vi "e.gate HighSpeedPort CodeDataType.vi"(8 "error in (no error)":errorcluster, 9 "Precision":i32, 10 "Value":dbl, 11 "TransferDataType":T1) -> (0 "error out":errorcluster, 1 "ByteCount":i32, 2 "DataTypeString":string, 3 "Binary data out":u8[](array[numeric]))   [LabVIEW 2016]
doc: "This vi codes a numeric value to a binary array with the right data type.\nData types are coded with fixed indexes.\n\nAlso some other useful information's are available."
uses:
  e.gate Data Type.ctl
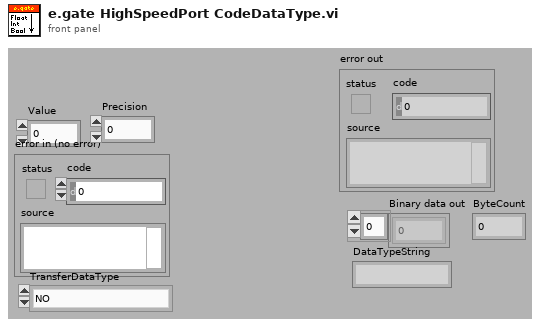
[diagram p1: front panel]
types:
  T1 = typedef "e.gate Data Type.ctl" = enum16{"NO", "BOOL", "SINT8", "USINT8", "SINT16", "USINT16", "SINT32", "USINT32", "FLOAT", "SET8", "SET16", "SET32", "DOUBLE", "SINT64", "USINT64", "SET64"}
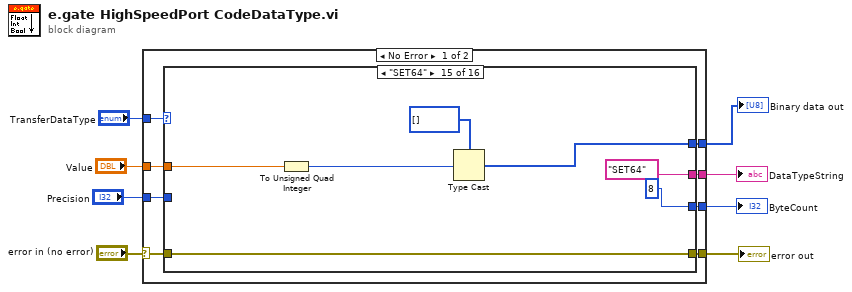
[diagram p0: block diagram]
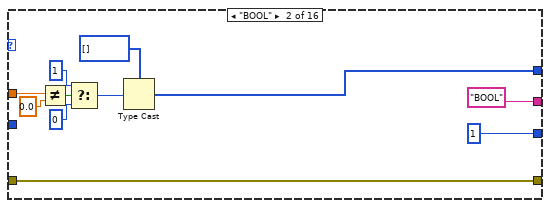
[diagram p3: hidden frame]
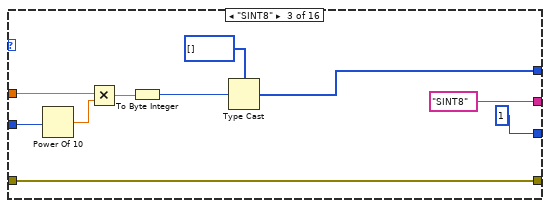
[diagram p4: hidden frame]
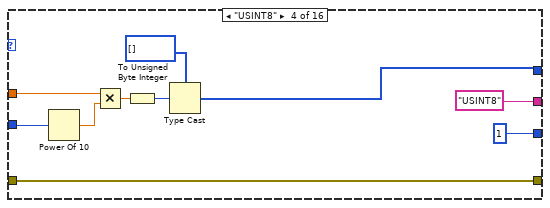
[diagram p5: hidden frame]
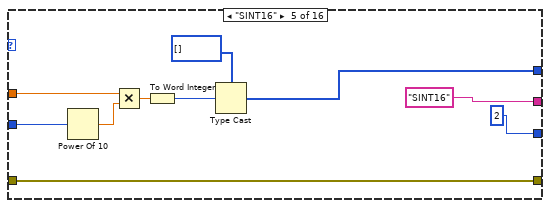
[diagram p6: hidden frame]
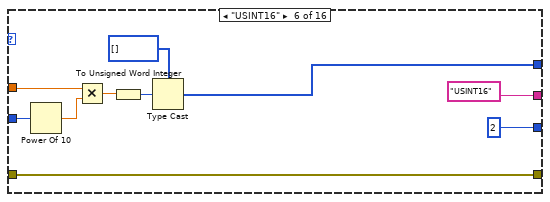
[diagram p7: hidden frame]
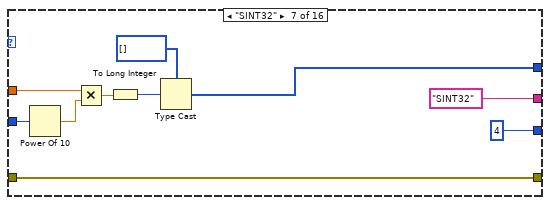
[diagram p8: hidden frame]
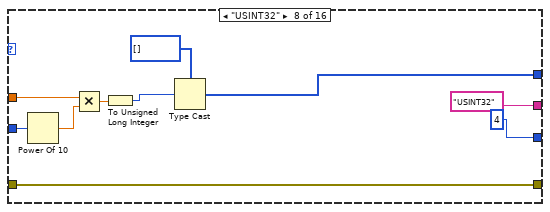
[diagram p9: hidden frame]
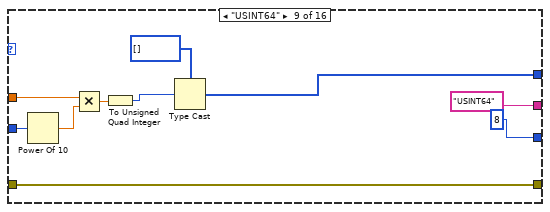
[diagram p10: hidden frame]
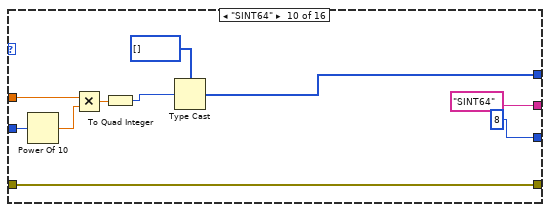
[diagram p11: hidden frame]
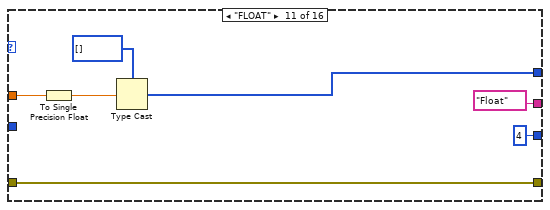
[diagram p12: hidden frame]
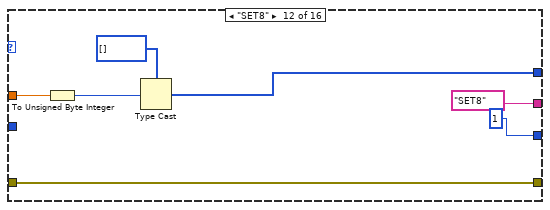
[diagram p13: hidden frame]
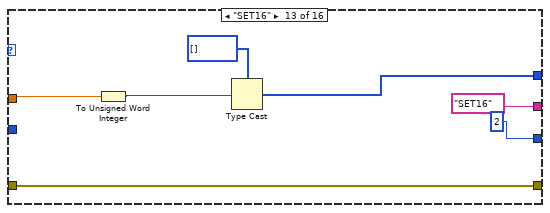
[diagram p14: hidden frame]
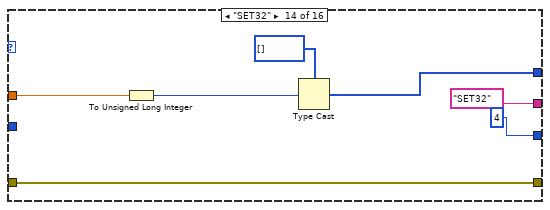
[diagram p15: hidden frame]
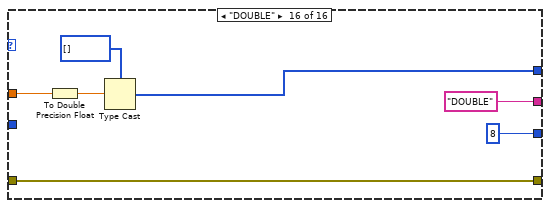
[diagram p16: hidden frame]
diagram:
  n1 = case shown="No Error" "error in (no error)" {
    selector: "error in (no error)" -> [w10 w151]
    tunnel: [w16 w151] -> w8
    tunnel: [w15 _] -> w7
    tunnel: [w14 _] -> w6
    tunnel: "TransferDataType" -> [w13 _]
    tunnel: "Value" -> [w12 _]
    tunnel: [w11 _] -> w4
    tunnel: "Precision" -> [w9 _]
    frame No Error {
      n2 = case shown="\"SET64\"" w13 {
        tunnel: [_ "BOOL" "SINT8" "USINT8" "SINT16" "USINT16" "SINT32" "USINT32" "USINT64" "SINT64" "Float" "SET8" "SET16" "SET32" "SET64" "DOUBLE"] -> w14
        tunnel: w12 -> [_ w23 w31 w41 w51 w61 w71 w81 w91 w101 w113 w119 w123 w130 w137 w148]
        tunnel: [_ i16 1 ("Precision") 1 1 ("Precision") 2 ("Precision") 2 ("Precision") 4 ("Precision") 4 ("Precision") 8 ("Precision") 8 ("Precision") 4 ("Precision") 1 ("Precision") 2 ("Precision") 4 ("Precision") 8 ("Precision") i16 8 ("Precision")] -> w15
        tunnel: [_ w18 w35 w45 w55 w64 w74 w84 w94 w104 w109 w116 w125 w132 w139 w144] -> w11
        tunnel: w10 -> [w17 w21 w34 w44 w54 w66 w76 w86 w96 w106 w112 w120 w127 w134 w141 w147]
        tunnel: [w17 w21 w34 w44 w54 w66 w76 w86 w96 w106 w112 w120 w127 w134 w141 w147] -> w16
        tunnel: w9 -> [_ _ w33 w42 w52 w62 w72 w82 w92 w102 _ _ _ _ _ _]
        frame "NO", Default {
        }
        frame "BOOL" {
          n3 = Not Equal?(x=w23, y=0.0) -> (x != y?=w24:bool)
          n4 = Select(t=u8 1, s=w24, f=u8 0) -> (s? t:f=w20:u8)
          n5 = Type Cast(type=u8[] [] ("Binary data out"), x=w20) -> (*(type *) &x=w18:u8[])
        }
        frame "SINT8" {
          n6 = Power Of 10(x=w33) -> (10^x=w32:dbl)
          n7 = Multiply(x=w31, y=w32) -> (x*y=w30:dbl)
          n8 = To Byte Integer(number=w30) -> (8bit integer=w29:i8)
          n9 = Type Cast(type=u8[] [] ("Binary data out"), x=w29) -> (*(type *) &x=w35:u8[])
        }
        frame "USINT8" {
          n10 = Power Of 10(x=w42) -> (10^x=w43:dbl)
          n11 = Multiply(x=w41, y=w43) -> (x*y=w40:dbl)
          n12 = To Unsigned Byte Integer(number=w40) -> (unsigned 8bit integer=w39:u8)
          n13 = Type Cast(type=u8[] [] ("Binary data out"), x=w39) -> (*(type *) &x=w45:u8[])
        }
        frame "SINT16" {
          n14 = Power Of 10(x=w52) -> (10^x=w53:dbl)
          n15 = Multiply(x=w51, y=w53) -> (x*y=w50:dbl)
          n16 = To Word Integer(number=w50) -> (16bit integer=w49:i16)
          n17 = Type Cast(type=u8[] [] ("Binary data out"), x=w49) -> (*(type *) &x=w55:u8[])
        }
        frame "USINT16" {
          n18 = Power Of 10(x=w62) -> (10^x=w63:dbl)
          n19 = Multiply(x=w61, y=w63) -> (x*y=w60:dbl)
          n20 = To Unsigned Word Integer(number=w60) -> (unsigned 16bit integer=w59:u16)
          n21 = Type Cast(type=u8[] [] ("Binary data out"), x=w59) -> (*(type *) &x=w64:u8[])
        }
        frame "SINT32" {
          n22 = Power Of 10(x=w72) -> (10^x=w73:dbl)
          n23 = Multiply(x=w71, y=w73) -> (x*y=w70:dbl)
          n24 = To Long Integer(number=w70) -> (32bit integer=w69:i32)
          n25 = Type Cast(type=u8[] [] ("Binary data out"), x=w69) -> (*(type *) &x=w74:u8[])
        }
        frame "USINT32" {
          n26 = Power Of 10(x=w82) -> (10^x=w83:dbl)
          n27 = Multiply(x=w81, y=w83) -> (x*y=w80:dbl)
          n28 = To Unsigned Long Integer(number=w80) -> (unsigned 32bit integer=w79:u32)
          n29 = Type Cast(type=u8[] [] ("Binary data out"), x=w79) -> (*(type *) &x=w84:u8[])
        }
        frame "USINT64" {
          n30 = Power Of 10(x=w92) -> (10^x=w93:dbl)
          n31 = Multiply(x=w91, y=w93) -> (x*y=w90:dbl)
          n32 = To Unsigned Quad Integer(1:w90) -> (0:w89:u64)
          n33 = Type Cast(type=u8[] [] ("Binary data out"), x=w89) -> (*(type *) &x=w94:u8[])
        }
        frame "SINT64" {
          n34 = Power Of 10(x=w102) -> (10^x=w103:dbl)
          n35 = Multiply(x=w101, y=w103) -> (x*y=w100:dbl)
          n36 = To Quad Integer(1:w100) -> (0:w99:i64)
          n37 = Type Cast(type=u8[] [] ("Binary data out"), x=w99) -> (*(type *) &x=w104:u8[])
        }
        frame "FLOAT" {
          n38 = To Single Precision Float(number=w113) -> (single precision float=w110:sgl)
          n39 = Type Cast(type=u8[] [] ("Binary data out"), x=w110) -> (*(type *) &x=w109:u8[])
        }
        frame "SET8" {
          n40 = To Unsigned Byte Integer(number=w119) -> (unsigned 8bit integer=w117:u8)
          n41 = Type Cast(type=u8[] [] ("Binary data out"), x=w117) -> (*(type *) &x=w116:u8[])
        }
        frame "SET16" {
          n42 = To Unsigned Word Integer(number=w123) -> (unsigned 16bit integer=w124:u16)
          n43 = Type Cast(type=u8[] [] ("Binary data out"), x=w124) -> (*(type *) &x=w125:u8[])
        }
        frame "SET32" {
          n44 = To Unsigned Long Integer(number=w130) -> (unsigned 32bit integer=w131:u32)
          n45 = Type Cast(type=u8[] [] ("Binary data out"), x=w131) -> (*(type *) &x=w132:u8[])
        }
        frame "SET64" {
          n46 = To Unsigned Quad Integer(1:w137) -> (0:w138:u64)
          n47 = Type Cast(type=u8[] [] ("Binary data out"), x=w138) -> (*(type *) &x=w139:u8[])
        }
        frame "DOUBLE" {
          n48 = To Double Precision Float(number=w148) -> (double precision float=w145:dbl)
          n49 = Type Cast(type=u8[] [] ("Binary data out"), x=w145) -> (*(type *) &x=w144:u8[])
        }
      }
    }
    frame Error {
    }
  }
  "error out" <- w8
  "Binary data out" <- w4
  "ByteCount" <- w7
  "DataTypeString" <- w6
